vi "Kill Process by PID.vi"(8 "error in (no error)":errorcluster, 11 "PID":i32) -> (0 "error out":errorcluster)   [LabVIEW 2018]
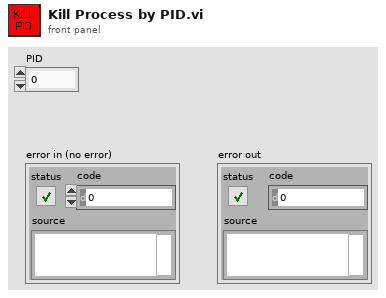
[diagram p1: front panel]
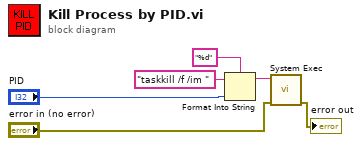
[diagram p0: block diagram]
diagram:
  n1 = Format Into String(format string="%d", initial string="taskkill /f /im ", "PID") -> (resulting string=w4:string)  [unwired: 1 in, 1 out]
  n2 = call <vilib>:"System Exec.vi"("error in (no error)"="error in (no error)", "command line"=w4) -> ("error out"=→"error out":errorcluster)  [unwired: 6 in, 3 out]
